vi "Close.vi"(8 "error in (no error)":errorcluster, 11 "Plugin in":refnum<class "Generic Plugin.lvclass">) -> (0 "error out":errorcluster)   [LabVIEW 2020, in "RxnRover.lvlib" / "Generic Plugin.lvclass"]
doc: "Shuts down the plugin server, destroying references and queues it generated. This will not destroy externally set references and queues."
uses:
  Generic Plugin.lvclass/Generic Plugin.ctl
  Generic Plugin.lvclass
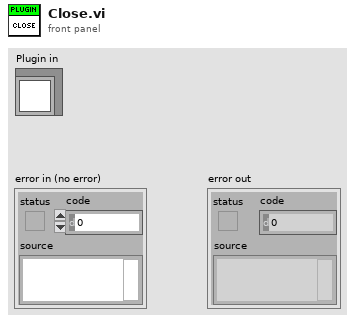
[diagram p1: front panel]
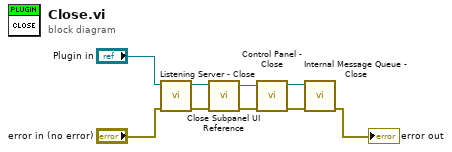
[diagram p0: block diagram]
diagram:
  n1 = call-dynamic "Listening Server - Close.vi"("error in (no error)"="error in (no error)", "Plugin in"="Plugin in") -> ("error out"=w8:errorcluster, "Plugin out"=w5:refnum<class "Generic Plugin.lvclass">)  [unwired: 8 in]
  n2 = call "Close Subpanel UI Reference.vi"("Plugin in"=w5, "error in (no error)"=w8) -> ("Plugin out"=w4:refnum<class "Generic Plugin.lvclass">, "error out"=w7:errorcluster)  [unwired: 1 in]
  n3 = call "Control Panel - Close.vi"("error in (no error)"=w7, "Plugin Server in"=w4) -> ("error out"=w6:errorcluster, "Plugin Server out"=w3:refnum<class "Generic Plugin.lvclass">)  [unwired: 8 in]
  n4 = call "Internal Message Queue - Close.vi"("error in (no error)"=w6, "Plugin in"=w3) -> ("error out"=→"error out":errorcluster)  [unwired: 8 in, 1 out]
